vi "Test DIO tasks.vi"() -> ()   [LabVIEW 2012]
uses:
  Controls/DIOTypedef.ctl
panel:
  in  "DIO Cluster":T1
  in  "stop":bool
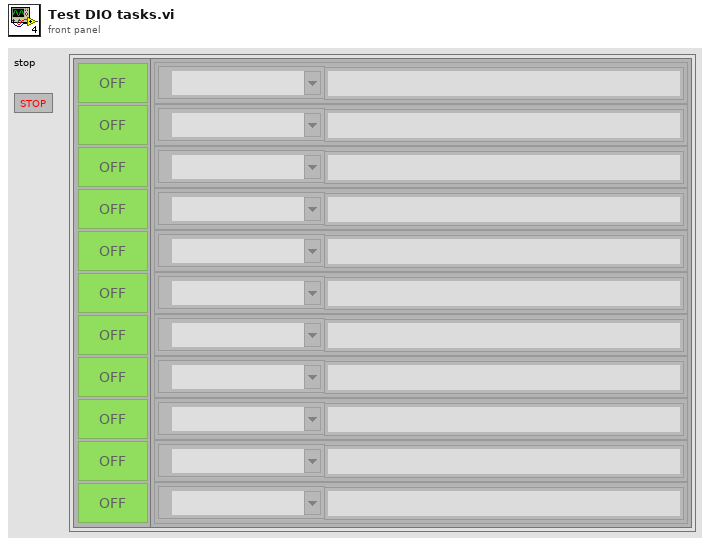
[diagram p1: front panel]
types:
  T1 = typedef "DIOTypedef.ctl" = cluster{"DIO Booleans":bool[], "DIO Channel Array":cluster{"Channel Name":string, "DIO lines":tag}[]}
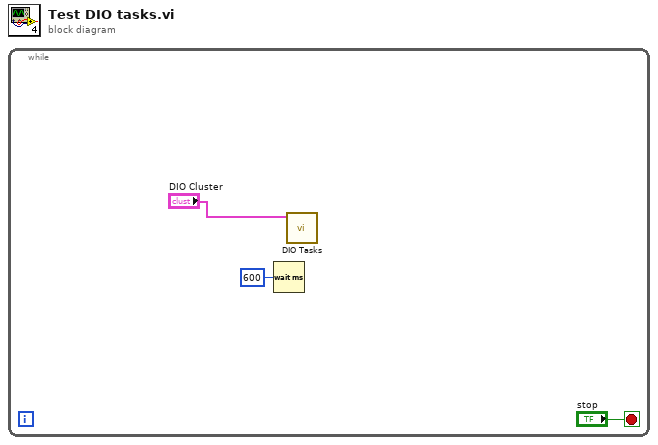
[diagram p0: block diagram]
diagram:
  n1 = while {
    stop <- "stop" stop-if-true
    n2 = Wait (ms)(milliseconds to wait=u32 600) -> ()  [unwired: 1 out]
    n3 = call "DIO Tasks.vi"("DIO Cluster"="DIO Cluster") -> ()  [unwired: 10 in, 1 out]
  }
